vi "曲线111.vi"() -> ()   [LabVIEW 2020]
uses:
  <vilib>/Utility/config.llb/NI_LVConfig.lvlib
  Global_Variable/A131258.vi
  Global_Variable/Global.vi
panel:
  in  "报表":string[][](table)=[["mm"], ["mm/s"]]
  in  "判定结果 3":bool[][](array[boolean])=[[TRUE]]
  in  "选项卡控件 2":enum32{"左工位压装曲线", "右工位压装曲线 ", "参数查看"}(tab)
  out "左压装下限":dbl format="%#.2f"
  out "左压装上限":dbl format="%#.2f"
  out "左下限2":dbl format="%#.2f"
  out "左上限2":dbl format="%#.2f"
  out "左下限1":dbl format="%#.2f"
  out "左上限1":dbl format="%#.2f"
  out "压装最大位移(mm)":dbl
  out "判定结果":bool
  out "力位移曲线":cluster{dbl[], dbl[]}[](graph)
  out "位移区间最大压力(KN)":dbl
  out "位移区间最小压力(KN)":dbl
  out "右位移下限":dbl format="%#.2f"
  out "右位移上限":dbl format="%#.2f"
  out "右下限2":dbl format="%#.2f"
  out "右上限2":dbl format="%#.2f"
  out "右下限1":dbl format="%#.2f"
  out "右上限1":dbl format="%#.2f"
  out "压装最大位移(mm) 2":dbl
  out "判定结果 2":bool
  out "力位移曲线 2":cluster{dbl[], dbl[]}[](graph)
  out "位移区间最大压力(KN) 2":dbl
  out "位移区间最小压力(KN) 2":dbl
  in  "删除":bool
  in  "确定":bool
  in  "添加":bool
  in  "退出":bool
  in  "更新":bool
  in  "产品型号":string(combo)
  in  "选项卡控件 3":enum32{"左工位参数", "右工位参数", "产品管理"}(tab)
  in  "左工位坐标轴参数":string[][](table)=[["mm"], ["mm/s"]]
  in  "左工位判定框参数":string[][](table)=[["mm"], ["mm/s"]]
  in  "左工位结果判定参数":string[][](table)=[["mm"], ["mm/s"]]
  in  "右工位结果判定参数":string[][](table)=[["mm"], ["mm/s"]]
  in  "右工位判定框参数":string[][](table)=[["mm"], ["mm/s"]]
  in  "右工位坐标轴参数":string[][](table)=[["mm"], ["mm/s"]]
  in  "请输入添加的产品名称":string
  in  "请选择要删除的产品":string(combo)
  # "180上下柱管总成装配"
  # "上限"
  # "下限"
  # "上限"
  # "下限"
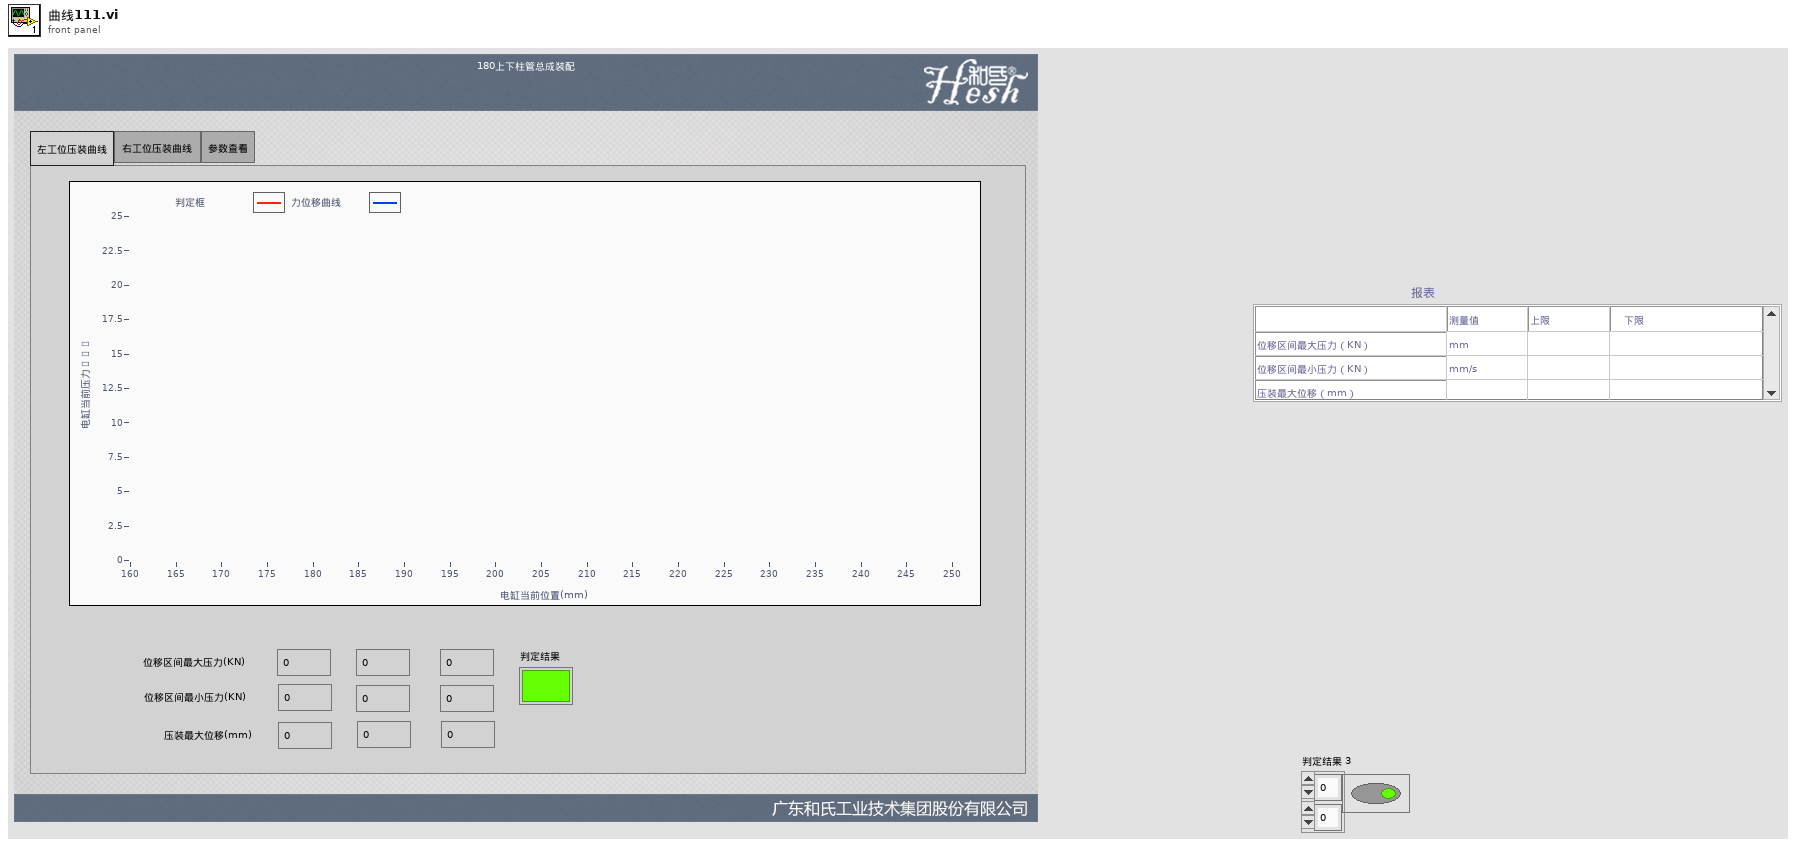
[diagram p1: front panel]
types:
  T1 = typedef "NI_LVConfig.lvlib/Config Data RefNum.ctl" = refnum<k1>
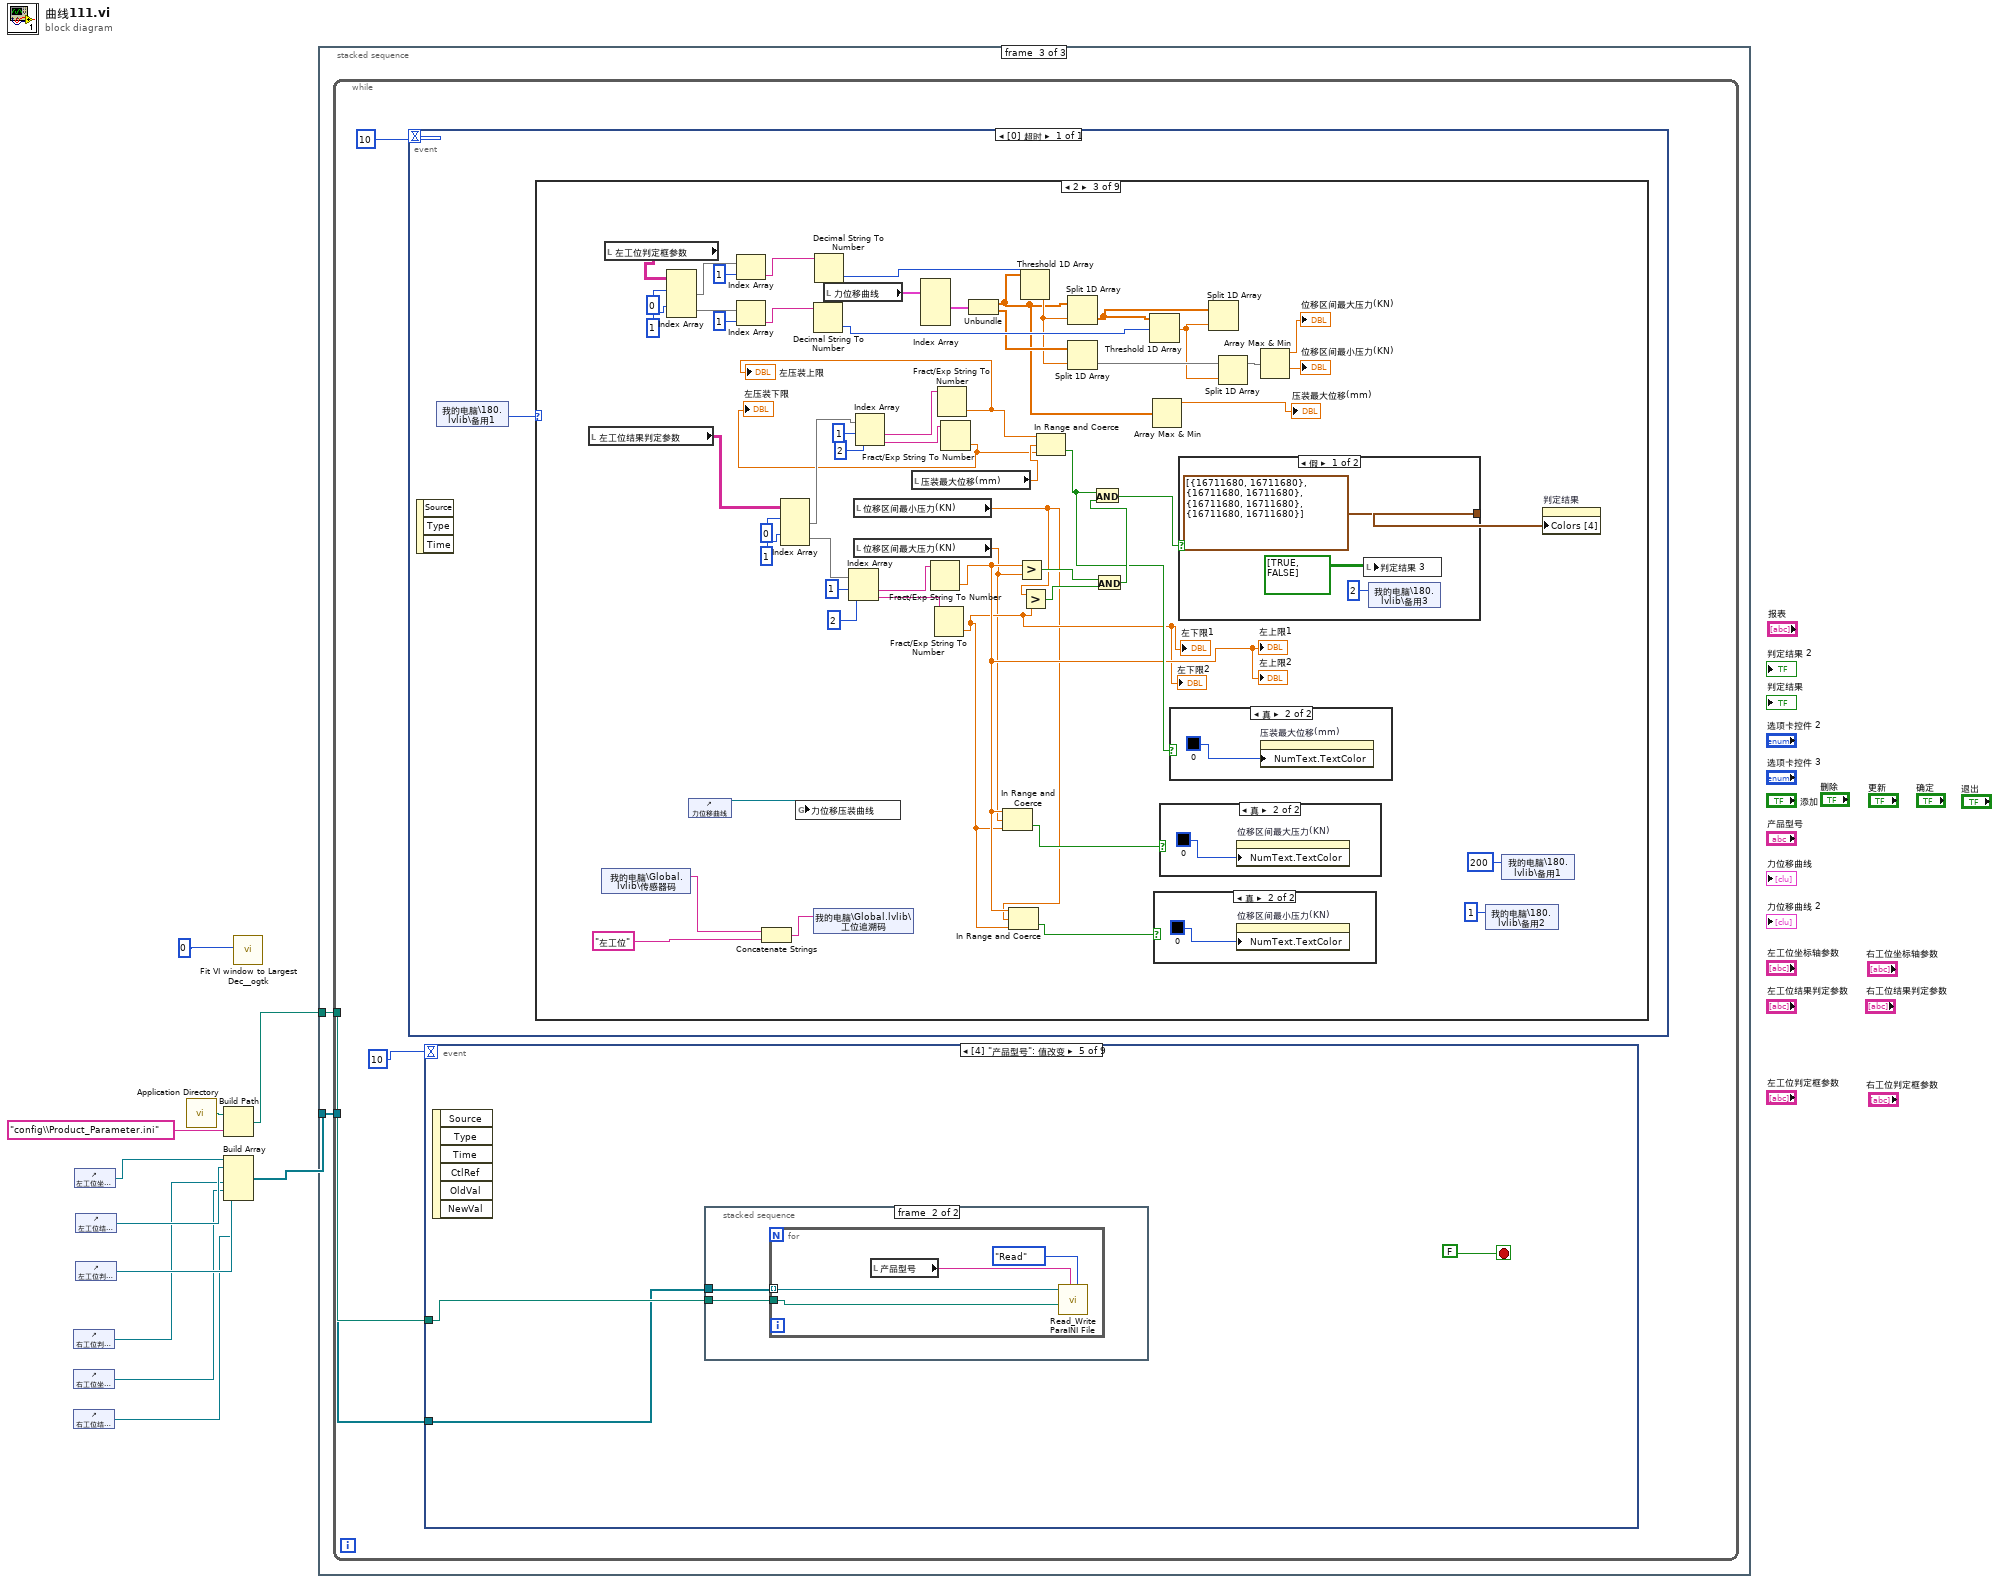
[diagram p0: block diagram]
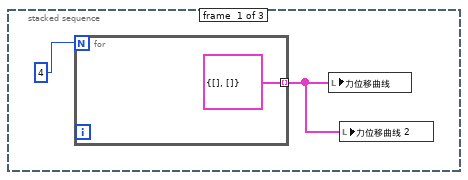
[diagram p2: hidden frame]
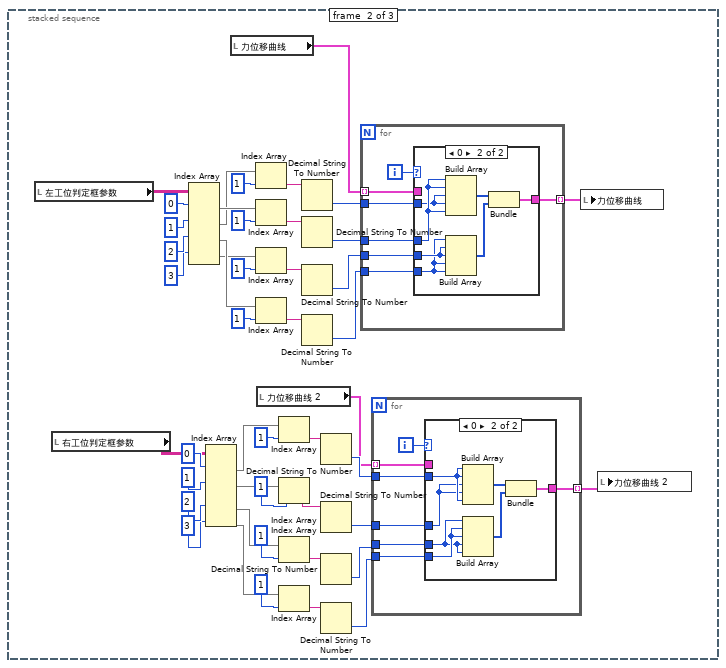
[diagram p3: hidden frame]
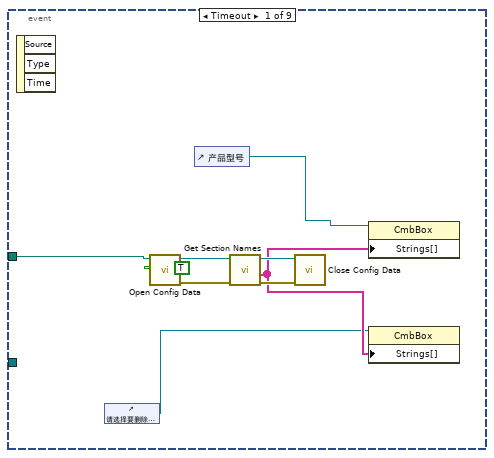
[diagram p6: hidden frame]
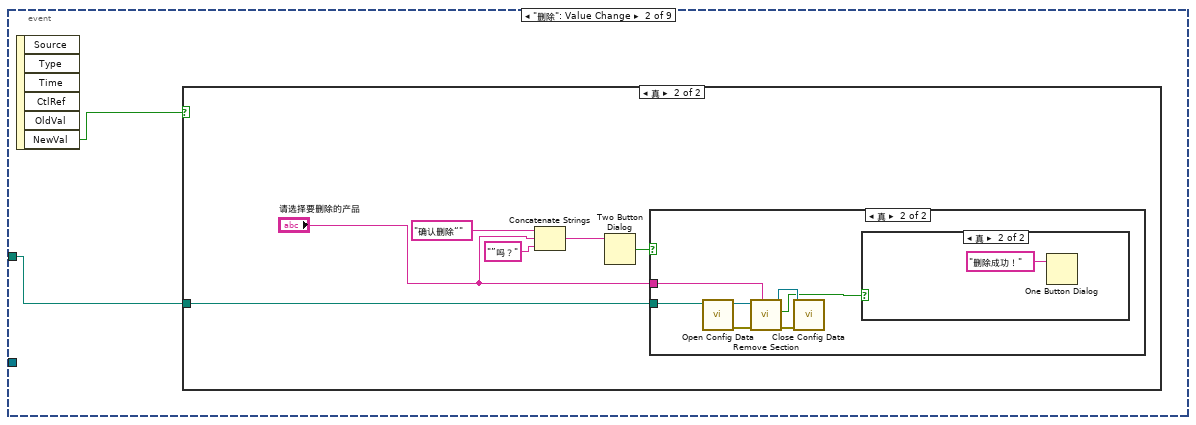
[diagram p7: hidden frame]
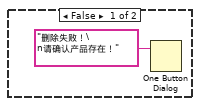
[diagram p10: hidden frame]
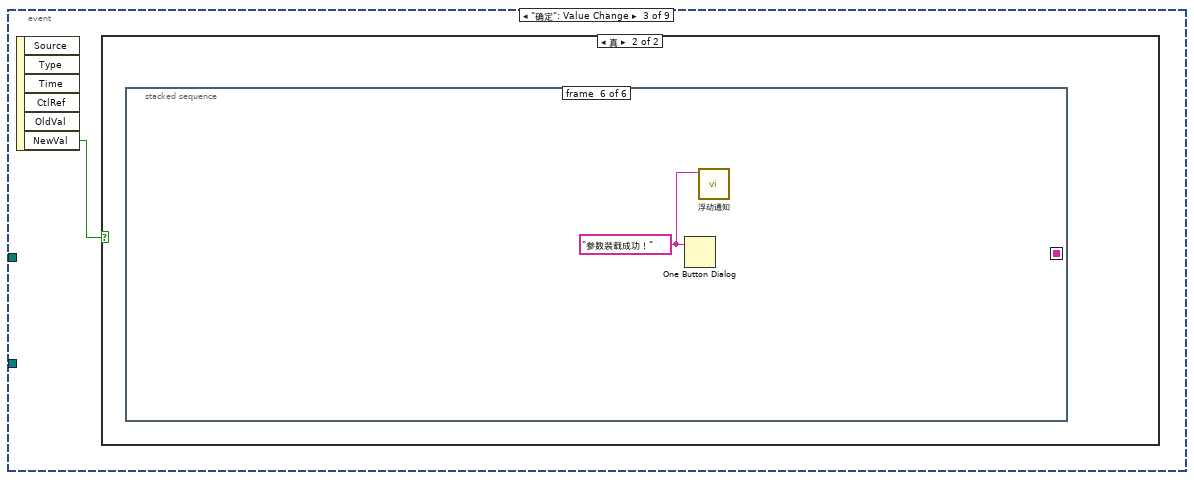
[diagram p11: hidden frame]
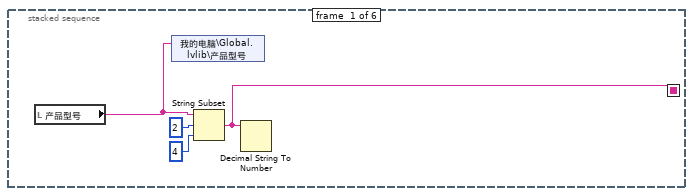
[diagram p13: hidden frame]
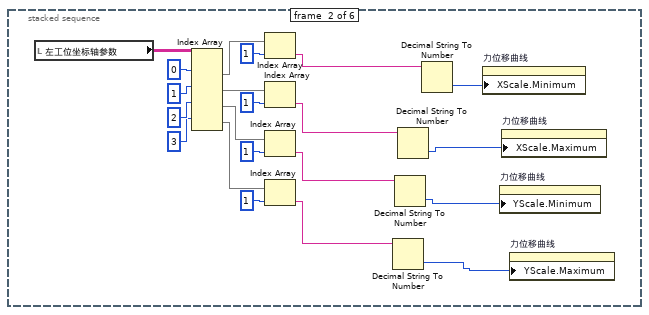
[diagram p14: hidden frame]
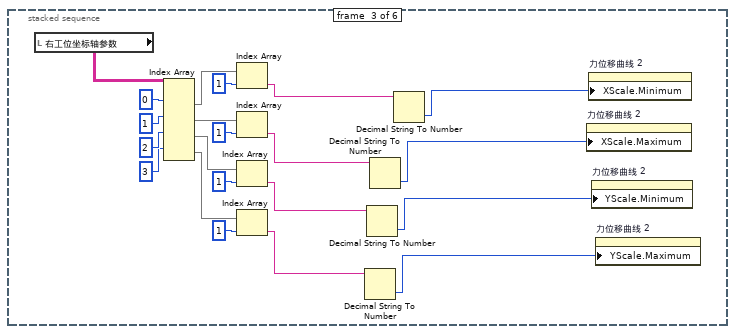
[diagram p15: hidden frame]
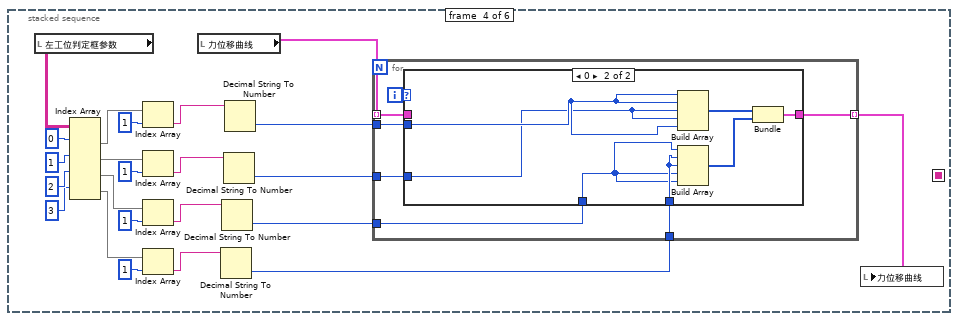
[diagram p16: hidden frame]
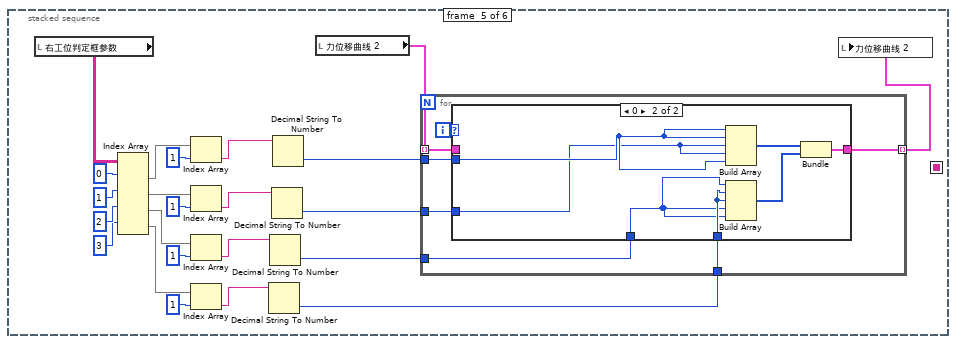
[diagram p18: hidden frame]
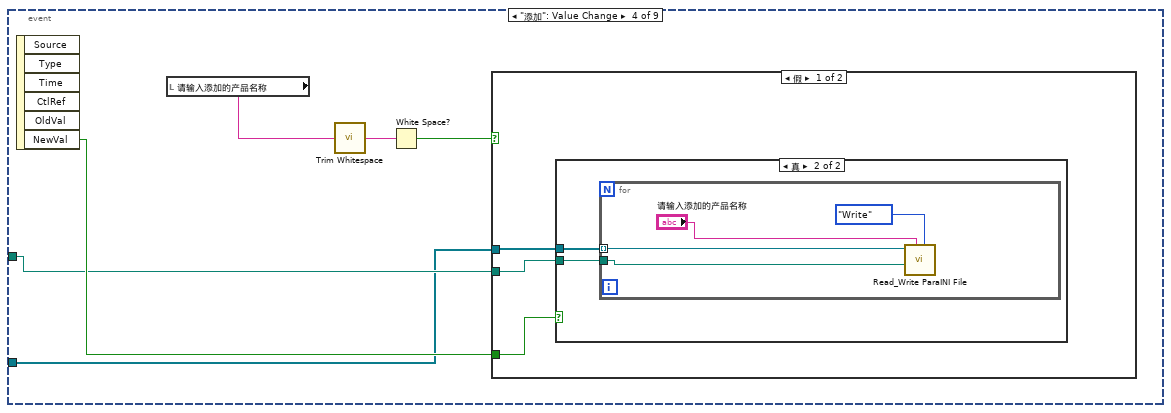
[diagram p20: hidden frame]
diagram:
  n1 = control-ref of="右工位判定框参数"() -> (w3:refnum<vi>)
  n2 = control-ref of="右工位坐标轴参数"() -> (w2:refnum<vi>)
  n3 = control-ref of="右工位结果判定参数"() -> (w1:refnum<vi>)
  n4 = control-ref of="左工位坐标轴参数"() -> (w6:refnum<vi>)
  n5 = control-ref of="左工位结果判定参数"() -> (w5:refnum<vi>)
  n6 = control-ref of="左工位判定框参数"() -> (w4:refnum<vi>)
  n7 = call <vilib>:"Application Directory.vi"() -> ("Application Directory"=w11:path)
  n8 = Build Path(base path=w11, name or relative path="config\\Product_Parameter.ini" ("名称或相对路径")) -> (appended path=w8:path)
  n9 = Build Array(w6, w5, w4, w3, w2, w1) -> (w7:refnum<vi>[])
  n10 = call <userlib>:"Fit VI window to Largest Dec__ogtk.vi"("border spacing (2 px)"=0) -> ()  [unwired: 5 in, 2 out]
  n11 = stacked-sequence {
    tunnel: w8 -> [_ _ w92]
    tunnel: w7 -> [_ _ w91]
    frame #0 {
      n12 = for {
        N: 4 -> [_]
        tunnel: [cluster{dbl[], dbl[]} {[], []}] -> w12 mode=indexing
      }
      n13 = local write "力位移曲线"(w12) -> ()
      n14 = local write "力位移曲线 2"(w12) -> ()
    }
    frame #1 {
      n15 = local read "左工位判定框参数"() -> (w15:string[][])
      n16 = local read "右工位判定框参数"() -> (w18:string[][])
      n17 = Index Array(array=w15, index (row) #1=0 ("索引 (行)"), index (row) #2=1 ("索引 (行)"), index (row) #3=2 ("索引 (行)"), index (row) #4=3 ("索引 (行)")) -> (element #1=w56:string[], element #2=w51:string[], element #3=w50:string[], element #4=w49:string[])  [unwired: 4 in]
      n18 = Index Array(array=w18, index (row) #1=0 ("索引 (行)"), index (row) #2=1 ("索引 (行)"), index (row) #3=2 ("索引 (行)"), index (row) #4=3 ("索引 (行)")) -> (element #1=w34:string[], element #2=w29:string[], element #3=w28:string[], element #4=w27:string[])  [unwired: 4 in]
      n19 = local read "力位移曲线"() -> (w39:cluster{dbl[], dbl[]}[])
      n20 = Index Array(array=w51, index=1 ("索引")) -> (element=w43:string)
      n21 = Index Array(array=w56, index=1 ("索引")) -> (element=w44:string)
      n22 = Index Array(array=w49, index=1 ("索引")) -> (element=w41:string)
      n23 = Index Array(array=w50, index=1 ("索引")) -> (element=w42:string)
      n24 = local read "力位移曲线 2"() -> (w17:cluster{dbl[], dbl[]}[])
      n25 = Index Array(array=w34, index=1 ("索引")) -> (element=w22:string)
      n26 = Index Array(array=w29, index=1 ("索引")) -> (element=w21:string)
      n27 = Index Array(array=w28, index=1 ("索引")) -> (element=w20:string)
      n28 = Index Array(array=w27, index=1 ("索引")) -> (element=w19:string)
      n29 = Decimal String To Number(string=w43) -> (number=w47:i32)  [unwired: 2 in, 1 out]
      n30 = Decimal String To Number(string=w44) -> (number=w48:i32)  [unwired: 2 in, 1 out]
      n31 = Decimal String To Number(string=w41) -> (number=w46:i32)  [unwired: 2 in, 1 out]
      n32 = Decimal String To Number(string=w42) -> (number=w45:i32)  [unwired: 2 in, 1 out]
      n33 = Decimal String To Number(string=w22) -> (number=w26:i32)  [unwired: 2 in, 1 out]
      n34 = Decimal String To Number(string=w21) -> (number=w25:i32)  [unwired: 2 in, 1 out]
      n35 = Decimal String To Number(string=w20) -> (number=w23:i32)  [unwired: 2 in, 1 out]
      n36 = Decimal String To Number(string=w19) -> (number=w24:i32)  [unwired: 2 in, 1 out]
      n37 = for {
        tunnel: [w82] -> w40 mode=indexing
        tunnel: w39 -> [w81] mode=indexing
        tunnel: w48 -> [w79]
        tunnel: w47 -> [w78]
        tunnel: w46 -> [w77]
        tunnel: w45 -> [w76]
        i -> [w80]
        n38 = case shown="0" w80 {
          tunnel: [w83 w88] -> w82
          tunnel: w81 -> [w83 _]
          tunnel: w79 -> [_ w87]
          tunnel: w78 -> [_ w86]
          tunnel: w77 -> [_ w85]
          tunnel: w76 -> [_ w84]
          frame Default {
          }
          frame 0 {
            n39 = Build Array(w87, w87, w86, w86, w87) -> (w89:i32[])
            n40 = Build Array(w84, w85, w85, w84, w84) -> (w90:i32[])
            n41 = Bundle(w89, w90) -> (w88:cluster{i32[], i32[]})  [unwired: 1 in]
          }
        }
      }
      n42 = for {
        tunnel: [w67] -> w16 mode=indexing
        tunnel: w17 -> [w66] mode=indexing
        tunnel: w26 -> [w64]
        tunnel: w25 -> [w63]
        tunnel: w24 -> [w62]
        tunnel: w23 -> [w61]
        i -> [w65]
        n43 = case shown="0" w65 {
          tunnel: [w68 w73] -> w67
          tunnel: w66 -> [w68 _]
          tunnel: w64 -> [_ w72]
          tunnel: w63 -> [_ w71]
          tunnel: w62 -> [_ w70]
          tunnel: w61 -> [_ w69]
          frame Default {
          }
          frame 0 {
            n44 = Build Array(w72, w72, w71, w71, w72) -> (w74:i32[])
            n45 = Build Array(w69, w70, w70, w69, w69) -> (w75:i32[])
            n46 = Bundle(w74, w75) -> (w73:cluster{i32[], i32[]})  [unwired: 1 in]
          }
        }
      }
      n47 = local write "力位移曲线"(w40) -> ()
      n48 = local write "力位移曲线 2"(w16) -> ()
    }
    frame #2 {
      n49 = while {
        tunnel: w92 -> [w94]
        tunnel: w91 -> [w93]
        stop <- FALSE stop-if-true
        n50 = event shown="[0] 超时" {
          selector: _ -> [_]
          dyn-events: _ -> [_]
          timeout: 10 -> [_]
          event Timeout {
            n51 = event-data() -> ()  [unwired: 1 in, 3 out]
            n52 = shared-variable "我的电脑\\180.lvlib\\备用1"() -> (w306:u16)  [unwired: 1 in, 1 out]
            n53 = case shown="2" w306 {
              frame 0, Default {
              }
              frame 1 {
                n54 = shared-variable "我的电脑\\180.lvlib\\备用2"() -> (w307:u16)  [unwired: 1 in, 1 out]
                n55 = case shown="1" w307 {
                  frame 0, Default {
                  }
                  frame 1 {
                    n56 = local read "力位移曲线"() -> (w309:cluster{dbl[], dbl[]}[])
                    n57 = for {
                      tunnel: [w313] -> w308 mode=indexing
                      tunnel: w309 -> [w312] mode=indexing
                      i -> [w311]
                      n58 = case shown="1" w311 {
                        tunnel: [w314 w318] -> w313
                        tunnel: w312 -> [w314 w317]
                        frame Default {
                        }
                        frame 1 {
                          n59 = Unbundle(w317) -> (w322:dbl[], w321:dbl[])
                          n60 = shared-variable "我的电脑\\180.lvlib\\电缸位移"() -> (w324:sgl[])  [unwired: 1 in, 1 out]
                          n61 = shared-variable "我的电脑\\180.lvlib\\电缸压力"() -> (w326:sgl[])  [unwired: 1 in, 1 out]
                          n62 = Index Array(array=w324, index=4) -> (element=w315:sgl)
                          n63 = Index Array(array=w326, index=4) -> (element=w316:sgl)
                          n64 = Build Array (concatenate)(w322, w315) -> (w320:dbl[])
                          n65 = Build Array (concatenate)(w321, w316) -> (w319:dbl[])
                          n66 = Bundle(w320, w319) -> (w318:cluster{dbl[], dbl[]})  [unwired: 1 in]
                        }
                      }
                    }
                    n67 = property on="选项卡控件 2" class="TabCtl (严格)"("Value"=enum32{"左工位压装曲线", "右工位压装曲线 ", "参数查看"}."左工位压装曲线" ("选项卡控件 2")) -> ()  [unwired: 2 in, 2 out]
                    n68 = local write "力位移曲线"(w308) -> ()
                  }
                  frame 2 {
                    n69 = local read "力位移曲线 2"() -> (w328:cluster{dbl[], dbl[]}[])
                    n70 = for {
                      tunnel: [w332] -> w329 mode=indexing
                      tunnel: w328 -> [w331] mode=indexing
                      i -> [w330]
                      n71 = case shown="1" w330 {
                        tunnel: [w333 w337] -> w332
                        tunnel: w331 -> [w333 w336]
                        frame Default {
                        }
                        frame 1 {
                          n72 = Unbundle(w336) -> (w341:dbl[], w340:dbl[])
                          n73 = shared-variable "我的电脑\\180.lvlib\\电缸位移"() -> (w343:sgl[])  [unwired: 1 in, 1 out]
                          n74 = shared-variable "我的电脑\\180.lvlib\\电缸压力"() -> (w345:sgl[])  [unwired: 1 in, 1 out]
                          n75 = Index Array(array=w343, index=4) -> (element=w334:sgl)
                          n76 = Index Array(array=w345, index=4) -> (element=w335:sgl)
                          n77 = Build Array (concatenate)(w341, w334) -> (w339:dbl[])
                          n78 = Build Array (concatenate)(w340, w335) -> (w338:dbl[])
                          n79 = Bundle(w339, w338) -> (w337:cluster{dbl[], dbl[]})  [unwired: 1 in]
                        }
                      }
                    }
                    n80 = property on="选项卡控件 2" class="TabCtl (严格)"("Value"=enum32{"左工位压装曲线", "右工位压装曲线 ", "参数查看"}."右工位压装曲线 " ("选项卡控件 2")) -> ()  [unwired: 2 in, 2 out]
                    n81 = local write "力位移曲线 2"(w329) -> ()
                  }
                }
              }
              frame 2 {
                n82 = local read "左工位结果判定参数"() -> (w373:string[][])
                n83 = shared-variable "我的电脑\\Global.lvlib\\传感器码"() -> (w346:string)  [unwired: 1 in, 1 out]
                n84 = local read "左工位判定框参数"() -> (w401:string[][])
                n85 = Index Array(array=w401, index (row) #1=0 ("索引 (行)"), index (row) #2=1 ("索引 (行)")) -> (element #1=w397:string[], element #2=w398:string[])  [unwired: 2 in]
                n86 = control-ref of="力位移曲线"() -> (w351:refnum<vi>)
                n87 = Index Array(array=w397, index=1 ("索引")) -> (element=w399:string)
                n88 = Index Array(array=w398, index=1 ("索引")) -> (element=w400:string)
                n89 = Concatenate Strings(w346, "左工位" ("字符串")) -> (w347:string)
                n90 = Index Array(array=w373, index (row) #1=0 ("索引 (行)"), index (row) #2=1 ("索引 (行)")) -> (element #1=w374:string[], element #2=w379:string[])  [unwired: 2 in]
                n91 = global write "A131258.vi" "力位移压装曲线"(w351) -> ()
                n92 = Decimal String To Number(string=w400) -> (number=w402:i32)  [unwired: 2 in, 1 out]
                n93 = shared-variable "我的电脑\\Global.lvlib\\工位追溯码"(w347) -> ()  [unwired: 1 in, 1 out]
                n94 = Decimal String To Number(string=w399) -> (number=w382:i32)  [unwired: 2 in, 1 out]
                n95 = local read "力位移曲线"() -> (w396:cluster{dbl[], dbl[]}[])
                n96 = Index Array(array=w379, index #1=1 ("索引"), index #2=2 ("索引")) -> (element #1=w367:string, element #2=w366:string)
                n97 = local read "位移区间最小压力(KN)"() -> (w352:dbl)
                n98 = local read "位移区间最大压力(KN)"() -> (w353:dbl)
                n99 = Index Array(array=w374, index #1=1 ("索引"), index #2=2 ("索引")) -> (element #1=w369:string, element #2=w368:string)
                n100 = local read "压装最大位移(mm)"() -> (w370:dbl)
                n101 = Index Array(array=w396) -> (element #2=w395:cluster{dbl[], dbl[]})  [unwired: 4 in, 3 out]
                n102 = Fract/Exp String To Number(string=w367) -> (number=w355:dbl)  [unwired: 3 in, 1 out]
                "左上限1" <- w355
                "左上限2" <- w355
                n103 = Fract/Exp String To Number(string=w366) -> (number=w354:dbl)  [unwired: 3 in, 1 out]
                "左下限1" <- w354
                "左下限2" <- w354
                n104 = Fract/Exp String To Number(string=w369) -> (number=w360:dbl)  [unwired: 3 in, 1 out]
                "左压装上限" <- w360
                n105 = Fract/Exp String To Number(string=w368) -> (number=w359:dbl)  [unwired: 3 in, 1 out]
                "左压装下限" <- w359
                n106 = Unbundle(w395) -> (w380:dbl[], w394:dbl[])
                n107 = In Range and Coerce(upper limit=w355, x=w353, lower limit=w354) -> (In Range?=w357:bool)  [unwired: 1 out]
                n108 = In Range and Coerce(upper limit=w355, x=w352, lower limit=w354) -> (In Range?=w356:bool)  [unwired: 1 out]
                n109 = Greater?(x=w355, y=w353) -> (0:w365:bool)
                n110 = Threshold 1D Array(2:w382, 3:w380) -> (0:w393:dbl)  [unwired: 1 in]
                n111 = Greater?(x=w352, y=w354) -> (0:w364:bool)
                n112 = In Range and Coerce(upper limit=w360, x=w370, lower limit=w359) -> (In Range?=w358:bool)  [unwired: 1 out]
                n113 = Split 1D Array(array=w380, index=w393) -> (second subarray=w391:dbl[])  [unwired: 1 out]
                n114 = Split 1D Array(array=w394, index=w393) -> (second subarray=w392:dbl[])  [unwired: 1 out]
                n115 = And(x=w365, y=w364) -> (x .and. y?=w363:bool)
                n116 = And(x=w358, y=w363) -> (x .and. y?=w362:bool)
                n117 = Threshold 1D Array(2:w402, 3:w391) -> (0:w390:dbl)  [unwired: 1 in]
                n118 = Array Max & Min(array=w380) -> (max value=→"压装最大位移(mm)":dbl)  [unwired: 3 out]
                n119 = case shown="真" w356 {
                  frame False {
                    n120 = property on="位移区间最小压力(KN)" class="DigNum (严格)"("NumText.TextColor"=u32 16716800) -> ()  [unwired: 2 in, 2 out]
                  }
                  frame True {
                    n121 = property on="位移区间最小压力(KN)" class="DigNum (严格)"("NumText.TextColor"=u32 0) -> ()  [unwired: 2 in, 2 out]
                  }
                }
                n122 = case shown="真" w357 {
                  frame False {
                    n123 = property on="位移区间最大压力(KN)" class="DigNum (严格)"("NumText.TextColor"=u32 16716800) -> ()  [unwired: 2 in, 2 out]
                  }
                  frame True {
                    n124 = property on="位移区间最大压力(KN)" class="DigNum (严格)"("NumText.TextColor"=u32 0) -> ()  [unwired: 2 in, 2 out]
                  }
                }
                n125 = case shown="真" w358 {
                  frame False {
                    n126 = property on="压装最大位移(mm)" class="DigNum (严格)"("NumText.TextColor"=u32 16716800) -> ()  [unwired: 2 in, 2 out]
                  }
                  frame True {
                    n127 = property on="压装最大位移(mm)" class="DigNum (严格)"("NumText.TextColor"=u32 0) -> ()  [unwired: 2 in, 2 out]
                  }
                }
                n128 = case shown="假" w362 {
                  tunnel: [cluster{u32, u32}[] [{16711680, 16711680}, {16711680, 16711680}, {16711680, 16711680}, {16711680, 16711680}] cluster{u32, u32}[] [{6618880, 6618880}, {6618880, 6618880}, {6618880, 6618880}, {6618880, 6618880}]] -> w361
                  frame False {
                    n129 = local write "判定结果 3"(bool[][] [[TRUE, FALSE]] ("判定结果")) -> ()
                    n130 = shared-variable "我的电脑\\180.lvlib\\备用3"(u16 2 ("备用1")) -> ()  [unwired: 1 in, 1 out]
                  }
                  frame True {
                    n131 = local write "判定结果 3"(bool[][] [[TRUE, TRUE]] ("判定结果")) -> ()
                    n132 = shared-variable "我的电脑\\180.lvlib\\备用3"(u16 1 ("备用1")) -> ()  [unwired: 1 in, 1 out]
                  }
                }
                n133 = Split 1D Array(array=w391, index=w390) -> ()  [unwired: 2 out]
                n134 = Split 1D Array(array=w392, index=w390) -> (first subarray=w389:dbl[])  [unwired: 1 out]
                n135 = Array Max & Min(array=w389) -> (max value=→"位移区间最大压力(KN)":dbl, min value=→"位移区间最小压力(KN)":dbl)  [unwired: 2 out]
                n136 = shared-variable "我的电脑\\180.lvlib\\备用2"(u16 1 ("备用1")) -> ()  [unwired: 1 in, 1 out]
                n137 = shared-variable "我的电脑\\180.lvlib\\备用1"(u16 200 ("备用1")) -> ()  [unwired: 1 in, 1 out]
                n138 = property on="判定结果" class="Bool (严格)"("Colors [4]"=w361) -> ()  [unwired: 2 in, 2 out]
              }
              frame 3 {
                n139 = local read "右工位判定框参数"() -> (w457:string[][])
                n140 = local read "右工位结果判定参数"() -> (w450:string[][])
                n141 = Index Array(array=w450, index (row) #1=0 ("索引 (行)"), index (row) #2=1 ("索引 (行)")) -> (element #1=w451:string[], element #2=w452:string[])  [unwired: 2 in]
                n142 = Index Array(array=w457, index (row) #1=0 ("索引 (行)"), index (row) #2=1 ("索引 (行)")) -> (element #1=w467:string[], element #2=w468:string[])  [unwired: 2 in]
                n143 = local read "位移区间最小压力(KN) 2"() -> (w431:dbl)
                n144 = local read "位移区间最大压力(KN) 2"() -> (w432:dbl)
                n145 = Index Array(array=w452, index #1=1 ("索引"), index #2=2 ("索引")) -> (element #1=w448:string, element #2=w447:string)
                n146 = Index Array(array=w467, index=1 ("索引")) -> (element=w469:string)
                n147 = Index Array(array=w468, index=1 ("索引")) -> (element=w470:string)
                n148 = control-ref of="力位移曲线 2"() -> (w420:refnum<vi>)
                n149 = Fract/Exp String To Number(string=w447) -> (number=w433:dbl)  [unwired: 3 in, 1 out]
                "右下限1" <- w433
                "右下限2" <- w433
                n150 = Fract/Exp String To Number(string=w448) -> (number=w434:dbl)  [unwired: 3 in, 1 out]
                "右上限1" <- w434
                "右上限2" <- w434
                n151 = Index Array(array=w451, index #1=1 ("索引"), index #2=2 ("索引")) -> (element #1=w449:string, element #2=w446:string)
                n152 = Decimal String To Number(string=w470) -> (number=w471:i32)  [unwired: 2 in, 1 out]
                n153 = Decimal String To Number(string=w469) -> (number=w455:i32)  [unwired: 2 in, 1 out]
                n154 = local read "力位移曲线 2"() -> (w458:cluster{dbl[], dbl[]}[])
                n155 = local read "压装最大位移(mm) 2"() -> (w445:dbl)
                n156 = Fract/Exp String To Number(string=w449) -> (number=w440:dbl)  [unwired: 3 in, 1 out]
                "右位移上限" <- w440
                n157 = Fract/Exp String To Number(string=w446) -> (number=w439:dbl)  [unwired: 3 in, 1 out]
                "右位移下限" <- w439
                n158 = global write "A131258.vi" "力位移压装曲线"(w420) -> ()
                n159 = Greater Or Equal?(x=w434, y=w432) -> (x >= y?=w438:bool)
                n160 = Greater Or Equal?(x=w431, y=w433) -> (x >= y?=w443:bool)
                n161 = Index Array(array=w458) -> (element #2=w466:cluster{dbl[], dbl[]})  [unwired: 4 in, 3 out]
                n162 = In Range and Coerce(upper limit=w440, x=w445, lower limit=w439) -> (In Range?=w437:bool)  [unwired: 1 out]
                n163 = Unbundle(w466) -> (w453:dbl[], w465:dbl[])
                n164 = And(x=w438, y=w443) -> (x .and. y?=w444:bool)
                n165 = And(x=w437, y=w444) -> (x .and. y?=w442:bool)
                n166 = In Range and Coerce(upper limit=w434, x=w431, lower limit=w433) -> (In Range?=w436:bool)  [unwired: 1 out]
                n167 = In Range and Coerce(upper limit=w434, x=w432, lower limit=w433) -> (In Range?=w435:bool)  [unwired: 1 out]
                n168 = Threshold 1D Array(2:w455, 3:w453) -> (0:w456:dbl)  [unwired: 1 in]
                n169 = Split 1D Array(array=w453, index=w456) -> (second subarray=w463:dbl[])  [unwired: 1 out]
                n170 = Split 1D Array(array=w465, index=w456) -> (second subarray=w464:dbl[])  [unwired: 1 out]
                n171 = case shown="假" w442 {
                  tunnel: [cluster{u32, u32}[] [{16711680, 16711680}, {16711680, 16711680}, {16711680, 16711680}, {16711680, 16711680}] cluster{u32, u32}[] [{6618880, 6618880}, {6618880, 6618880}, {6618880, 6618880}, {6618880, 6618880}]] -> w441
                  frame False {
                    n172 = shared-variable "我的电脑\\180.lvlib\\备用3"(u16 2 ("备用1")) -> ()  [unwired: 1 in, 1 out]
                    n173 = local write "判定结果 3"(bool[][] [[TRUE, FALSE]] ("判定结果")) -> ()
                  }
                  frame True {
                    n174 = shared-variable "我的电脑\\180.lvlib\\备用3"(u16 1 ("备用1")) -> ()  [unwired: 1 in, 1 out]
                    n175 = local write "判定结果 3"(bool[][] [[TRUE, TRUE]] ("判定结果")) -> ()
                  }
                }
                n176 = case shown="真" w435 {
                  frame False {
                    n177 = property on="位移区间最大压力(KN) 2" class="DigNum (严格)"("NumText.TextColor"=u32 16720402) -> ()  [unwired: 2 in, 2 out]
                  }
                  frame True {
                    n178 = property on="位移区间最大压力(KN) 2" class="DigNum (严格)"("NumText.TextColor"=u32 0) -> ()  [unwired: 2 in, 2 out]
                  }
                }
                n179 = case shown="假" w436 {
                  frame False {
                    n180 = property on="位移区间最小压力(KN) 2" class="DigNum (严格)"("NumText.TextColor"=u32 16720402) -> ()  [unwired: 2 in, 2 out]
                  }
                  frame True {
                    n181 = property on="位移区间最小压力(KN) 2" class="DigNum (严格)"("NumText.TextColor"=u32 0) -> ()  [unwired: 2 in, 2 out]
                  }
                }
                n182 = case shown="假" w437 {
                  frame False {
                    n183 = property on="压装最大位移(mm) 2" class="DigNum (严格)"("NumText.TextColor"=u32 16720402) -> ()  [unwired: 2 in, 2 out]
                  }
                  frame True {
                    n184 = property on="压装最大位移(mm) 2" class="DigNum (严格)"("NumText.TextColor"=u32 0) -> ()  [unwired: 2 in, 2 out]
                  }
                }
                n185 = Array Max & Min(array=w453) -> (max value=→"压装最大位移(mm) 2":dbl)  [unwired: 3 out]
                n186 = Threshold 1D Array(2:w471, 3:w463) -> (0:w462:dbl)  [unwired: 1 in]
                n187 = Split 1D Array(array=w463, index=w462) -> ()  [unwired: 2 out]
                n188 = Split 1D Array(array=w464, index=w462) -> (first subarray=w461:dbl[])  [unwired: 1 out]
                n189 = Array Max & Min(array=w461) -> (max value=→"位移区间最大压力(KN) 2":dbl, min value=→"位移区间最小压力(KN) 2":dbl)  [unwired: 2 out]
                n190 = shared-variable "我的电脑\\Global.lvlib\\传感器码"() -> (w415:string)  [unwired: 1 in, 1 out]
                n191 = shared-variable "我的电脑\\180.lvlib\\备用2"(u16 2 ("备用1")) -> ()  [unwired: 1 in, 1 out]
                n192 = shared-variable "我的电脑\\180.lvlib\\备用1"(u16 200 ("备用1")) -> ()  [unwired: 1 in, 1 out]
                n193 = Concatenate Strings(w415, "右工位" ("字符串")) -> (w416:string)
                n194 = property on="判定结果 2" class="Bool (严格)"("Colors [4]"=w441) -> ()  [unwired: 2 in, 2 out]
                n195 = shared-variable "我的电脑\\Global.lvlib\\工位追溯码"(w416) -> ()  [unwired: 1 in, 1 out]
              }
              frame 100 {
                n196 = stacked-sequence {
                  frame #0 {
                    w486 = cluster{u32, u32}[] [{12369084, 12369084}, {12369084, 12369084}, {12369084, 12369084}, {12369084, 12369084}]
                    w487 = u32 0
                    w488 = 0.0 ("压装最大位移(mm)")
                    n197 = local write "压装最大位移(mm)"(w488) -> ()
                    n198 = local write "位移区间最小压力(KN)"(w488) -> ()
                    n199 = local write "位移区间最大压力(KN)"(w488) -> ()
                    n200 = local write "压装最大位移(mm) 2"(w488) -> ()
                    n201 = local write "位移区间最小压力(KN) 2"(w488) -> ()
                    n202 = local write "位移区间最大压力(KN) 2"(w488) -> ()
                    n203 = for {
                      N: 4 -> [_]
                      tunnel: [cluster{dbl[], dbl[]} {[], []}] -> w489 mode=indexing
                    }
                    n204 = global read "Global.vi" "Result"() -> (w484:refnum<vi>)
                    n205 = property on="位移区间最大压力(KN) 2" class="DigNum (严格)"("NumText.TextColor"=w487) -> ()  [unwired: 2 in, 2 out]
                    n206 = property on="压装最大位移(mm) 2" class="DigNum (严格)"("NumText.TextColor"=w487) -> ()  [unwired: 2 in, 2 out]
                    n207 = property on="位移区间最小压力(KN) 2" class="DigNum (严格)"("NumText.TextColor"=w487) -> ()  [unwired: 2 in, 2 out]
                    n208 = property on="位移区间最大压力(KN)" class="DigNum (严格)"("NumText.TextColor"=w487) -> ()  [unwired: 2 in, 2 out]
                    n209 = property on="压装最大位移(mm)" class="DigNum (严格)"("NumText.TextColor"=w487) -> ()  [unwired: 2 in, 2 out]
                    n210 = property on="位移区间最小压力(KN)" class="DigNum (严格)"("NumText.TextColor"=w487) -> ()  [unwired: 2 in, 2 out]
                    n211 = property class="Tbl"(reference=w484, "Value"=string[][] []) -> ()  [unwired: 1 in, 2 out]
                    n212 = local write "力位移曲线"(w489) -> ()
                    n213 = local write "力位移曲线 2"(w489) -> ()
                    n214 = property on="判定结果" class="Bool (严格)"("Colors [4]"=w486) -> ()  [unwired: 2 in, 2 out]
                    n215 = property on="判定结果 2" class="Bool (严格)"("Colors [4]"=w486) -> ()  [unwired: 2 in, 2 out]
                  }
                  frame #1 {
                    n216 = local read "左工位判定框参数"() -> (w493:string[][])
                    n217 = local read "力位移曲线"() -> (w494:cluster{dbl[], dbl[]}[])
                    n218 = Index Array(array=w493, index (row) #1=0 ("索引 (行)"), index (row) #2=1 ("索引 (行)"), index (row) #3=2 ("索引 (行)"), index (row) #4=3 ("索引 (行)")) -> (element #1=w510:string[], element #2=w505:string[], element #3=w504:string[], element #4=w503:string[])  [unwired: 4 in]
                    n219 = Index Array(array=w505, index=1 ("索引")) -> (element=w497:string)
                    n220 = Index Array(array=w510, index=1 ("索引")) -> (element=w498:string)
                    n221 = Index Array(array=w503, index=1 ("索引")) -> (element=w495:string)
                    n222 = Index Array(array=w504, index=1 ("索引")) -> (element=w496:string)
                    n223 = Decimal String To Number(string=w497) -> (number=w501:i32)  [unwired: 2 in, 1 out]
                    n224 = Decimal String To Number(string=w498) -> (number=w502:i32)  [unwired: 2 in, 1 out]
                    n225 = Decimal String To Number(string=w495) -> (number=w500:i32)  [unwired: 2 in, 1 out]
                    n226 = Decimal String To Number(string=w496) -> (number=w499:i32)  [unwired: 2 in, 1 out]
                    n227 = for {
                      tunnel: [w521] -> w492 mode=indexing
                      tunnel: w494 -> [w520] mode=indexing
                      tunnel: w502 -> [w518]
                      tunnel: w501 -> [w517]
                      tunnel: w500 -> [w516]
                      tunnel: w499 -> [w515]
                      i -> [w519]
                      n228 = case shown="0" w519 {
                        tunnel: [w522 w527] -> w521
                        tunnel: w520 -> [w522 _]
                        tunnel: w518 -> [_ w526]
                        tunnel: w517 -> [_ w525]
                        tunnel: w516 -> [_ w524]
                        tunnel: w515 -> [_ w523]
                        frame Default {
                        }
                        frame 0 {
                          n229 = Build Array(w526, w526, w525, w525, w526) -> (w528:i32[])
                          n230 = Build Array(w523, w524, w524, w523, w523) -> (w529:i32[])
                          n231 = Bundle(w528, w529) -> (w527:cluster{i32[], i32[]})  [unwired: 1 in]
                        }
                      }
                    }
                    n232 = local write "力位移曲线"(w492) -> ()
                  }
                  frame #2 {
                    n233 = local read "右工位判定框参数"() -> (w530:string[][])
                    n234 = local read "力位移曲线 2"() -> (w532:cluster{dbl[], dbl[]}[])
                    n235 = Index Array(array=w530, index (row) #1=0 ("索引 (行)"), index (row) #2=1 ("索引 (行)"), index (row) #3=2 ("索引 (行)"), index (row) #4=3 ("索引 (行)")) -> (element #1=w548:string[], element #2=w543:string[], element #3=w542:string[], element #4=w541:string[])  [unwired: 4 in]
                    n236 = Index Array(array=w543, index=1 ("索引")) -> (element=w535:string)
                    n237 = Index Array(array=w548, index=1 ("索引")) -> (element=w536:string)
                    n238 = Index Array(array=w541, index=1 ("索引")) -> (element=w533:string)
                    n239 = Index Array(array=w542, index=1 ("索引")) -> (element=w534:string)
                    n240 = Decimal String To Number(string=w535) -> (number=w539:i32)  [unwired: 2 in, 1 out]
                    n241 = Decimal String To Number(string=w536) -> (number=w540:i32)  [unwired: 2 in, 1 out]
                    n242 = Decimal String To Number(string=w533) -> (number=w538:i32)  [unwired: 2 in, 1 out]
                    n243 = Decimal String To Number(string=w534) -> (number=w537:i32)  [unwired: 2 in, 1 out]
                    n244 = for {
                      tunnel: [w559] -> w531 mode=indexing
                      tunnel: w532 -> [w558] mode=indexing
                      tunnel: w540 -> [w556]
                      tunnel: w539 -> [w555]
                      tunnel: w538 -> [w554]
                      tunnel: w537 -> [w553]
                      i -> [w557]
                      n245 = case shown="0" w557 {
                        tunnel: [w560 w565] -> w559
                        tunnel: w558 -> [w560 _]
                        tunnel: w556 -> [_ w564]
                        tunnel: w555 -> [_ w563]
                        tunnel: w554 -> [_ w562]
                        tunnel: w553 -> [_ w561]
                        frame Default {
                        }
                        frame 0 {
                          n246 = Build Array(w564, w564, w563, w563, w564) -> (w566:i32[])
                          n247 = Build Array(w561, w562, w562, w561, w561) -> (w567:i32[])
                          n248 = Bundle(w566, w567) -> (w565:cluster{i32[], i32[]})  [unwired: 1 in]
                        }
                      }
                    }
                    n249 = local write "力位移曲线 2"(w531) -> ()
                  }
                }
              }
              frame 200 {
                n250 = shared-variable "我的电脑\\180.lvlib\\备用2"() -> (w571:u16)  [unwired: 1 in, 1 out]
                n251 = stacked-sequence {
                  frame #0 {
                    n252 = Wait (ms)(milliseconds to wait=u32 500 ("等待时间（毫秒）")) -> ()  [unwired: 1 out]
                    n253 = call "浮动通知.vi"("通知内容"="报表生成中" ("Status")) -> ()  [unwired: 11 in]
                  }
                  frame #1 {
                  }
                }
                n254 = case shown="2" w571 {
                  tunnel: [_ w572 w603] -> w569
                  frame 0, Default {
                  }
                  frame 1 {
                    n255 = local read "左下限2"() -> (w577:dbl)
                    n256 = local read "压装最大位移(mm)"() -> (w583:dbl)
                    n257 = local read "左压装上限"() -> (w576:dbl)
                    n258 = local read "左压装下限"() -> (w575:dbl)
                    n259 = local read "位移区间最小压力(KN)"() -> (w579:dbl)
                    n260 = local read "左上限2"() -> (w578:dbl)
                    n261 = local read "位移区间最大压力(KN)"() -> (w584:dbl)
                    n262 = Number To Fractional String(number=w579) -> (F-format string=w590:string)  [unwired: 3 in]
                    n263 = local read "左上限1"() -> (w581:dbl)
                    n264 = local read "左下限1"() -> (w580:dbl)
                    n265 = Number To Fractional String(number=w578) -> (F-format string=w589:string)  [unwired: 3 in]
                    n266 = Number To Fractional String(number=w575) -> (F-format string=w573:string)  [unwired: 3 in]
                    n267 = Number To Fractional String(number=w583) -> (F-format string=w582:string)  [unwired: 3 in]
                    n268 = Number To Fractional String(number=w576) -> (F-format string=w574:string)  [unwired: 3 in]
                    n269 = Number To Fractional String(number=w584) -> (F-format string=w593:string)  [unwired: 3 in]
                    n270 = Number To Fractional String(number=w577) -> (F-format string=w586:string)  [unwired: 3 in]
                    n271 = Number To Fractional String(number=w581) -> (F-format string=w592:string)  [unwired: 3 in]
                    n272 = Build Array(w590, w589, w586) -> (w588:string[])
                    n273 = Number To Fractional String(number=w580) -> (F-format string=w587:string)  [unwired: 3 in]
                    n274 = Build Array(w593, w592, w587) -> (w591:string[])
                    n275 = Build Array(w582, w574, w573) -> (w585:string[])
                    n276 = Build Array(w591, w588, w585) -> (w572:string[][])
                  }
                  frame 2 {
                    n277 = local read "右上限2"() -> (w598:dbl)
                    n278 = local read "压装最大位移(mm) 2"() -> (w596:dbl)
                    n279 = local read "右位移上限"() -> (w595:dbl)
                    n280 = local read "右位移下限"() -> (w594:dbl)
                    n281 = local read "位移区间最小压力(KN) 2"() -> (w599:dbl)
                    n282 = local read "右下限2"() -> (w597:dbl)
                    n283 = local read "位移区间最大压力(KN) 2"() -> (w602:dbl)
                    n284 = local read "右下限1"() -> (w600:dbl)
                    n285 = local read "右上限1"() -> (w601:dbl)
                    n286 = Number To Fractional String(number=w599) -> (F-format string=w612:string)  [unwired: 3 in]
                    n287 = Number To Fractional String(number=w598) -> (F-format string=w611:string)  [unwired: 3 in]
                    n288 = Number To Fractional String(number=w594) -> (F-format string=w604:string)  [unwired: 3 in]
                    n289 = Number To Fractional String(number=w596) -> (F-format string=w606:string)  [unwired: 3 in]
                    n290 = Number To Fractional String(number=w595) -> (F-format string=w605:string)  [unwired: 3 in]
                    n291 = Number To Fractional String(number=w602) -> (F-format string=w615:string)  [unwired: 3 in]
                    n292 = Number To Fractional String(number=w597) -> (F-format string=w608:string)  [unwired: 3 in]
                    n293 = Number To Fractional String(number=w601) -> (F-format string=w614:string)  [unwired: 3 in]
                    n294 = Build Array(w612, w611, w608) -> (w610:string[])
                    n295 = Number To Fractional String(number=w600) -> (F-format string=w609:string)  [unwired: 3 in]
                    n296 = Build Array(w615, w614, w609) -> (w613:string[])
                    n297 = Build Array(w606, w605, w604) -> (w607:string[])
                    n298 = Build Array(w613, w610, w607) -> (w603:string[][])
                  }
                }
                n299 = control-ref of="报表"() -> (w568:refnum<vi>)
                n300 = global write "Global.vi" "Result"(w568) -> ()
                n301 = shared-variable "我的电脑\\180.lvlib\\备用1"(u16 201 ("备用1")) -> ()  [unwired: 1 in, 1 out]
                n302 = local write "报表"(w569) -> ()
              }
              frame 201 {
                n303 = shared-variable "我的电脑\\Global.lvlib\\工位追溯码"() -> (w620:string)  [unwired: 1 in, 1 out]
                n304 = call "Report_A131258.vi"("文件重命名"=TRUE, "文件名称"=w620, "布尔数组"="判定结果 3") -> ()  [unwired: 8 in, 1 out]
                n305 = shared-variable "我的电脑\\180.lvlib\\备用1"(u16 0 ("备用1")) -> ()  [unwired: 1 in, 1 out]
                n306 = Wait (ms)(milliseconds to wait=u32 800 ("等待时间（毫秒）")) -> ()  [unwired: 1 out]
              }
              frame 1000 {
                n307 = stacked-sequence {
                  frame #0 {
                    n308 = shared-variable "我的电脑\\Global.lvlib\\传感器码"("" ("传感器码")) -> ()  [unwired: 1 in, 1 out]
                  }
                  frame #1 {
                    w626 = "请扫码！" ("通知内容")
                    n309 = call "浮动通知.vi"("通知内容"=w626) -> ()  [unwired: 11 in]
                    n310 = call "输入框.vi"("提示信息"=w626) -> ("条形码输出"=w625:string)
                    n311 = shared-variable "我的电脑\\Global.lvlib\\传感器码"(w625) -> ()  [unwired: 1 in, 1 out]
                    n312 = shared-variable "我的电脑\\180.lvlib\\备用1"(u16 1001 ("备用1")) -> ()  [unwired: 1 in, 1 out]
                  }
                }
              }
              frame 1001 {
                n313 = shared-variable "我的电脑\\Global.lvlib\\传感器码"() -> (w629:string)  [unwired: 1 in, 1 out]
                n314 = String Length(string=w629) -> (length=w628:i32)
                n315 = Greater?(x=w628, y=4) -> (0:w630:bool)
                n316 = case shown="真" w630 {
                  frame False {
                  }
                  frame True {
                    n317 = shared-variable "我的电脑\\180.lvlib\\备用1"(u16 1002 ("备用1")) -> ()  [unwired: 1 in, 1 out]
                  }
                }
              }
            }
          }
        }
        n318 = event shown="[4] \"产品型号\": 值改变" {
          selector: _ -> [_ _ _ _ _ _ _ _ _]
          dyn-events: _ -> [_ _ _ _ _ _ _ _ _]
          timeout: 10 -> [_ _ _ _ _ _ _ _ _]
          tunnel: w94 -> [w98 w108 _ w249 w268 _ w279 _ _]
          tunnel: w93 -> [_ _ _ w248 w267 _ w278 _ _]
          event Timeout {
            n319 = event-data() -> ()  [unwired: 1 in, 3 out]
            n320 = control-ref of="请选择要删除的产品"() -> (w99:refnum<vi>)
            n321 = call <vilib>:"Open Config Data.vi"("create file if necessary (T)"=TRUE, "configuration file path"=w98) -> ("error out"=w103:errorcluster, "refnum"=w102:T1)  [unwired: 7 in, 1 out]
            n322 = control-ref of="产品型号"() -> (w100:refnum<vi>)
            n323 = call <vilib>:"Get Section Names.vi"("error in (no error)"=w103, "refnum"=w102) -> ("error out"=w105:errorcluster, "section names"=w101:string[], "refnum out"=w104:T1)  [unwired: 7 in]
            n324 = call <vilib>:"Close Config Data.vi"("error in (no error)"=w105, "refnum"=w104) -> ()  [unwired: 8 in, 2 out]
            n325 = property on="属性节点" class="CmbBox"(reference=w100, "Strings[]"=w101) -> ()  [unwired: 1 in, 2 out]
            n326 = property on="属性节点" class="CmbBox"(reference=w99, "Strings[]"=w101) -> ()  [unwired: 1 in, 2 out]
          }
          event "删除": Value Change {
            n327 = event-data() -> ("NewVal"=w107:bool)  [unwired: 1 in, 5 out]
            n328 = case shown="真" w107 {
              tunnel: w108 -> [_ w110]
              frame False {
              }
              frame True {
                n329 = Concatenate Strings("确认删除“", "请选择要删除的产品", "”吗？") -> (w112:string)
                n330 = Two Button Dialog(message=w112) -> (T button?=w111:bool)  [unwired: 2 in]
                n331 = case shown="真" w111 {
                  tunnel: w110 -> [_ w116]
                  tunnel: "请选择要删除的产品" -> [_ w115]
                  frame False {
                  }
                  frame True {
                    n332 = call <vilib>:"Open Config Data.vi"("configuration file path"=w116) -> ("error out"=w118:errorcluster, "refnum"=w121:T1)  [unwired: 8 in, 1 out]
                    n333 = call <vilib>:"Remove Section.vi"("section"=w115, "error in (no error)"=w118, "refnum"=w121) -> ("error out"=w120:errorcluster, "section exists?"=w117:bool, "refnum out"=w119:T1)  [unwired: 6 in]
                    n334 = call <vilib>:"Close Config Data.vi"("error in (no error)"=w120, "refnum"=w119) -> ()  [unwired: 8 in, 2 out]
                    n335 = case shown="真" w117 {
                      frame False {
                        n336 = One Button Dialog(message="删除失败！\n请确认产品存在！" ("消息")) -> ()  [unwired: 1 in, 1 out]
                      }
                      frame True {
                        n337 = One Button Dialog(message="删除成功！" ("消息")) -> ()  [unwired: 1 in, 1 out]
                      }
                    }
                  }
                }
              }
            }
          }
          event "确定": Value Change {
            n338 = event-data() -> ("NewVal"=w124:bool)  [unwired: 1 in, 5 out]
            n339 = case shown="真" w124 {
              frame False {
              }
              frame True {
                n340 = stacked-sequence {
                  seq-local: [w125 _ _ _ _ _] -> [_ _ _ _ _ _]
                  frame #0 {
                    n341 = local read "产品型号"() -> (w128:string)
                    n342 = shared-variable "我的电脑\\Global.lvlib\\产品型号"(w128) -> ()  [unwired: 1 in, 1 out]
                    n343 = String Subset(string=w128, offset (0)=u16 2 ("偏移量(0)"), length (rest)=u16 4 ("长度（剩余）")) -> (substring=w125:string)
                    n344 = Decimal String To Number(string=w125) -> ()  [unwired: 2 in, 2 out]
                  }
                  frame #1 {
                    n345 = local read "左工位坐标轴参数"() -> (w129:string[][])
                    n346 = Index Array(array=w129, index (row) #1=0 ("索引 (行)"), index (row) #2=1 ("索引 (行)"), index (row) #3=2 ("索引 (行)"), index (row) #4=3 ("索引 (行)")) -> (element #1=w145:string[], element #2=w140:string[], element #3=w139:string[], element #4=w138:string[])  [unwired: 4 in]
                    n347 = Index Array(array=w145, index=1 ("索引")) -> (element=w137:string)
                    n348 = Index Array(array=w140, index=1 ("索引")) -> (element=w135:string)
                    n349 = Index Array(array=w139, index=1 ("索引")) -> (element=w134:string)
                    n350 = Index Array(array=w138, index=1 ("索引")) -> (element=w133:string)
                    n351 = Decimal String To Number(string=w133) -> (number=w130:i32)  [unwired: 2 in, 1 out]
                    n352 = Decimal String To Number(string=w134) -> (number=w131:i32)  [unwired: 2 in, 1 out]
                    n353 = Decimal String To Number(string=w135) -> (number=w132:i32)  [unwired: 2 in, 1 out]
                    n354 = Decimal String To Number(string=w137) -> (number=w136:i32)  [unwired: 2 in, 1 out]
                    n355 = property on="力位移曲线" class="XYGraph (严格)"("XScale.Minimum"=w136) -> ()  [unwired: 2 in, 2 out]
                    n356 = property on="力位移曲线" class="XYGraph (严格)"("YScale.Minimum"=w131) -> ()  [unwired: 2 in, 2 out]
                    n357 = property on="力位移曲线" class="XYGraph (严格)"("XScale.Maximum"=w132) -> ()  [unwired: 2 in, 2 out]
                    n358 = property on="力位移曲线" class="XYGraph (严格)"("YScale.Maximum"=w130) -> ()  [unwired: 2 in, 2 out]
                  }
                  frame #2 {
                    n359 = local read "右工位坐标轴参数"() -> (w154:string[][])
                    n360 = Index Array(array=w154, index (row) #1=0 ("索引 (行)"), index (row) #2=1 ("索引 (行)"), index (row) #3=2 ("索引 (行)"), index (row) #4=3 ("索引 (行)")) -> (element #1=w166:string[], element #2=w161:string[], element #3=w160:string[], element #4=w159:string[])  [unwired: 4 in]
                    n361 = Index Array(array=w166, index=1 ("索引")) -> (element=w158:string)
                    n362 = Index Array(array=w161, index=1 ("索引")) -> (element=w157:string)
                    n363 = Index Array(array=w160, index=1 ("索引")) -> (element=w156:string)
                    n364 = Index Array(array=w159, index=1 ("索引")) -> (element=w155:string)
                    n365 = Decimal String To Number(string=w155) -> (number=w150:i32)  [unwired: 2 in, 1 out]
                    n366 = Decimal String To Number(string=w156) -> (number=w151:i32)  [unwired: 2 in, 1 out]
                    n367 = Decimal String To Number(string=w157) -> (number=w152:i32)  [unwired: 2 in, 1 out]
                    n368 = Decimal String To Number(string=w158) -> (number=w153:i32)  [unwired: 2 in, 1 out]
                    n369 = property on="力位移曲线 2" class="XYGraph (严格)"("XScale.Maximum"=w152) -> ()  [unwired: 2 in, 2 out]
                    n370 = property on="力位移曲线 2" class="XYGraph (严格)"("XScale.Minimum"=w153) -> ()  [unwired: 2 in, 2 out]
                    n371 = property on="力位移曲线 2" class="XYGraph (严格)"("YScale.Minimum"=w151) -> ()  [unwired: 2 in, 2 out]
                    n372 = property on="力位移曲线 2" class="XYGraph (严格)"("YScale.Maximum"=w150) -> ()  [unwired: 2 in, 2 out]
                  }
                  frame #3 {
                    n373 = local read "左工位判定框参数"() -> (w180:string[][])
                    n374 = Index Array(array=w180, index (row) #1=0 ("索引 (行)"), index (row) #2=1 ("索引 (行)"), index (row) #3=2 ("索引 (行)"), index (row) #4=3 ("索引 (行)")) -> (element #1=w188:string[], element #2=w183:string[], element #3=w182:string[], element #4=w181:string[])  [unwired: 4 in]
                    n375 = Index Array(array=w188, index=1 ("索引")) -> (element=w175:string)
                    n376 = Index Array(array=w183, index=1 ("索引")) -> (element=w174:string)
                    n377 = Index Array(array=w182, index=1 ("索引")) -> (element=w173:string)
                    n378 = Index Array(array=w181, index=1 ("索引")) -> (element=w172:string)
                    n379 = local read "力位移曲线"() -> (w193:cluster{dbl[], dbl[]}[])
                    n380 = Decimal String To Number(string=w172) -> (number=w177:i32)  [unwired: 2 in, 1 out]
                    n381 = Decimal String To Number(string=w173) -> (number=w176:i32)  [unwired: 2 in, 1 out]
                    n382 = Decimal String To Number(string=w174) -> (number=w178:i32)  [unwired: 2 in, 1 out]
                    n383 = Decimal String To Number(string=w175) -> (number=w179:i32)  [unwired: 2 in, 1 out]
                    n384 = for {
                      tunnel: [w200] -> w171 mode=indexing
                      tunnel: w193 -> [w199] mode=indexing
                      tunnel: w179 -> [w197]
                      tunnel: w178 -> [w196]
                      tunnel: w177 -> [w195]
                      tunnel: w176 -> [w194]
                      i -> [w198]
                      n385 = case shown="0" w198 {
                        tunnel: [w201 w206] -> w200
                        tunnel: w199 -> [w201 _]
                        tunnel: w197 -> [_ w205]
                        tunnel: w196 -> [_ w204]
                        tunnel: w195 -> [_ w203]
                        tunnel: w194 -> [_ w202]
                        frame Default {
                        }
                        frame 0 {
                          n386 = Build Array(w205, w205, w204, w204, w205) -> (w207:i32[])
                          n387 = Build Array(w202, w203, w203, w202, w202) -> (w208:i32[])
                          n388 = Bundle(w207, w208) -> (w206:cluster{i32[], i32[]})  [unwired: 1 in]
                        }
                      }
                    }
                    n389 = local write "力位移曲线"(w171) -> ()
                  }
                  frame #4 {
                    n390 = local read "右工位判定框参数"() -> (w209:string[][])
                    n391 = Index Array(array=w209, index (row) #1=0 ("索引 (行)"), index (row) #2=1 ("索引 (行)"), index (row) #3=2 ("索引 (行)"), index (row) #4=3 ("索引 (行)")) -> (element #1=w227:string[], element #2=w222:string[], element #3=w221:string[], element #4=w220:string[])  [unwired: 4 in]
                    n392 = Index Array(array=w227, index=1 ("索引")) -> (element=w215:string)
                    n393 = Index Array(array=w222, index=1 ("索引")) -> (element=w214:string)
                    n394 = Index Array(array=w221, index=1 ("索引")) -> (element=w213:string)
                    n395 = Index Array(array=w220, index=1 ("索引")) -> (element=w212:string)
                    n396 = Decimal String To Number(string=w212) -> (number=w217:i32)  [unwired: 2 in, 1 out]
                    n397 = Decimal String To Number(string=w213) -> (number=w216:i32)  [unwired: 2 in, 1 out]
                    n398 = Decimal String To Number(string=w214) -> (number=w218:i32)  [unwired: 2 in, 1 out]
                    n399 = Decimal String To Number(string=w215) -> (number=w219:i32)  [unwired: 2 in, 1 out]
                    n400 = local read "力位移曲线 2"() -> (w210:cluster{dbl[], dbl[]}[])
                    n401 = for {
                      tunnel: [w238] -> w211 mode=indexing
                      tunnel: w210 -> [w237] mode=indexing
                      tunnel: w219 -> [w235]
                      tunnel: w218 -> [w234]
                      tunnel: w217 -> [w233]
                      tunnel: w216 -> [w232]
                      i -> [w236]
                      n402 = case shown="0" w236 {
                        tunnel: [w239 w244] -> w238
                        tunnel: w237 -> [w239 _]
                        tunnel: w235 -> [_ w243]
                        tunnel: w234 -> [_ w242]
                        tunnel: w233 -> [_ w241]
                        tunnel: w232 -> [_ w240]
                        frame Default {
                        }
                        frame 0 {
                          n403 = Build Array(w243, w243, w242, w242, w243) -> (w245:i32[])
                          n404 = Build Array(w240, w241, w241, w240, w240) -> (w246:i32[])
                          n405 = Bundle(w245, w246) -> (w244:cluster{i32[], i32[]})  [unwired: 1 in]
                        }
                      }
                    }
                    n406 = local write "力位移曲线 2"(w211) -> ()
                  }
                  frame #5 {
                    w247 = "参数装载成功！" ("消息")
                    n407 = One Button Dialog(message=w247) -> ()  [unwired: 1 in, 1 out]
                    n408 = call "浮动通知.vi"("通知内容"=w247) -> ()  [unwired: 11 in]
                  }
                }
              }
            }
          }
          event "添加": Value Change {
            n409 = event-data() -> ("NewVal"=w250:bool)  [unwired: 1 in, 5 out]
            n410 = local read "请输入添加的产品名称"() -> (w251:string)
            n411 = call <vilib>:"Trim Whitespace.vi"("string"=w251) -> ("trimmed string"=w252:string)  [unwired: 1 in]
            n412 = White Space?(1:w252) -> (0:w253:bool)
            n413 = case shown="假" w253 {
              tunnel: w248 -> [w256 _]
              tunnel: w250 -> [w255 _]
              tunnel: w249 -> [w254 _]
              frame False {
                n414 = case shown="真" w255 {
                  tunnel: w256 -> [_ w258]
                  tunnel: w254 -> [_ w257]
                  frame False {
                  }
                  frame True {
                    n415 = for {
                      tunnel: w258 -> [w261] mode=indexing
                      tunnel: w257 -> [w260]
                      n416 = call "Read_Write ParaINI File.vi"("Mode"=enum16{"Read", "Write"}."Write", "Section"="请输入添加的产品名称", "Filepath"=w260, "Ctl Refnum"=w261) -> ()  [unwired: 7 in, 1 out]
                    }
                  }
                }
              }
              frame True {
                w263 = 64 items=["None"=0, "Hand, Error, Stop"=16, "Question"=32, "Exclamation, Warning"=48, "Asterisk, Information"=64] ("icon")
                w264 = 0 items=["OK", "OKCancel", "AbortRetryIgnore", "YesNoCancel", "YesNo", "RetryCancel"] ("buttons")
                n417 = call "信息框（标题、文本、图标）.vi"("icon"=w263, "buttons"=w264, "caption"="添加失败", "text"="请输入产品名称!") -> ()  [unwired: 6 in, 2 out]
              }
            }
          }
          event "产品型号": Value Change {
            n418 = event-data() -> ()  [unwired: 1 in, 6 out]
            n419 = stacked-sequence {
              tunnel: w267 -> [_ w270]
              tunnel: w268 -> [_ w269]
              frame #0 {
              }
              frame #1 {
                n420 = for {
                  tunnel: w270 -> [w273] mode=indexing
                  tunnel: w269 -> [w272]
                  n421 = local read "产品型号"() -> (w271:string)
                  n422 = call "Read_Write ParaINI File.vi"("Mode"=enum16{"Read", "Write"}."Read", "Section"=w271, "Filepath"=w272, "Ctl Refnum"=w273) -> ()  [unwired: 7 in, 1 out]
                }
              }
            }
          }
          event "退出": Value Change {
            n423 = event-data() -> ()  [unwired: 1 in, 6 out]
            n424 = control-ref of="本VI"() -> (w277:refnum<vi>)
            n425 = invoke class="VI" method="FP.Close"(reference=w277) -> (reference out=w275:refnum<vi>, error out=w276:errorcluster)  [unwired: 2 in, 1 out]
            n426 = Close Reference(reference=w275, error in (no error)=w276) -> ()  [unwired: 1 out]
          }
          event "更新": Value Change {
            n427 = event-data() -> ("NewVal"=w280:bool)  [unwired: 1 in, 5 out]
            n428 = case shown="真" w280 {
              tunnel: w279 -> [_ w283]
              tunnel: w278 -> [_ w282]
              frame False {
              }
              frame True {
                n429 = for {
                  tunnel: w283 -> [w288]
                  tunnel: w282 -> [w287] mode=indexing
                  tunnel: [w286] -> w281
                  n430 = local read "产品型号"() -> (w290:string)
                  n431 = call "Read_Write ParaINI File.vi"("Mode"=enum16{"Read", "Write"}."Write", "Section"=w290, "Filepath"=w288, "Ctl Refnum"=w287) -> ("error out"=w286:errorcluster)  [unwired: 7 in]
                }
                n432 = case shown="无错误" w281 {
                  frame No Error {
                    n433 = call "浮动通知.vi"("通知内容"="更新成功！") -> ()  [unwired: 11 in]
                  }
                  frame Error {
                    n434 = call "浮动通知.vi"("通知内容"="更新失败！") -> ()  [unwired: 11 in]
                  }
                }
              }
            }
          }
          event "请输入添加的产品名称": Value Change {
            n435 = event-data() -> ("NewVal"=w291:string)  [unwired: 1 in, 5 out]
            n436 = control-ref of="产品型号"() -> (w292:refnum<vi>)
            n437 = property on="属性节点" class="CmbBox"(reference=w292) -> ("Strings[]"=w293:string[])  [unwired: 1 in, 2 out]
            n438 = for {
              tunnel: w291 -> [w294]
              tunnel: w293 -> [w295] mode=indexing
              n439 = Equal?(x=w294, y=w295) -> (x = y?=w296:bool)
              n440 = case shown="真" w296 {
                tunnel: w294 -> [_ w297]
                frame False {
                }
                frame True {
                  n441 = stacked-sequence {
                    tunnel: w297 -> [w303 _]
                    frame #0 {
                      w298 = 64 items=["None"=0, "Hand, Error, Stop"=16, "Question"=32, "Exclamation, Warning"=48, "Asterisk, Information"=64] ("icon")
                      w299 = 0 items=["OK", "OKCancel", "AbortRetryIgnore", "YesNoCancel", "YesNo", "RetryCancel"] ("buttons")
                      n442 = Concatenate Strings("已经存在产品”" ("text"), w303, "“\n请勿重复添加！" ("字符串")) -> (w301:string)
                      n443 = call "信息框（标题、文本、图标）.vi"("icon"=w298, "buttons"=w299, "caption"="产品重复", "text"=w301) -> ()  [unwired: 6 in, 2 out]
                    }
                    frame #1 {
                      n444 = local write "请输入添加的产品名称"("" ("请输入添加的产品名称")) -> ()
                    }
                  }
                }
              }
            }
          }
          event Panel Close {
            n445 = event-data() -> ()  [unwired: 1 in, 4 out]
          }
        }
      }
    }
  }
